vi "Number_Range.vi"() -> ()   [LabVIEW 2024]
panel:
  out "coerced(x)":dbl
  out "In Range?":bool
  in  "x":dbl
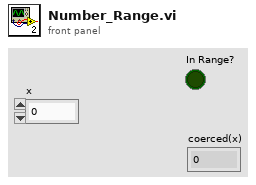
[diagram p1: front panel]
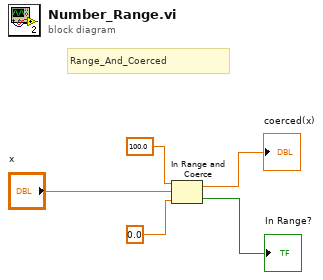
[diagram p0: block diagram]
diagram:
  # "Range_And_Coerced"
  n1 = In Range and Coerce(upper limit=100.0, x="x", lower limit=0.0) -> (coerced(x)=→"coerced(x)":dbl, In Range?=→"In Range?":bool)
